vi "Calculate Voltage Array.vi"(1 "I_peak":dbl, 2 "V_min":dbl, 3 "R_ref":dbl, 4 "Scale (True == Linear, False == Log)":bool, 5 "# pts":dbl, 6 "V_max":dbl) -> (0 "Voltage Array":dbl[](array[numeric]))   [LabVIEW 2020]
doc: "Calculate Voltage Array.vi outputs a double numeric array with an inputted number of voltages within an inputted range with an inputted spacing (linear or log). No more voltages are appended to the array when an inputted peak current can theoretically be reached."
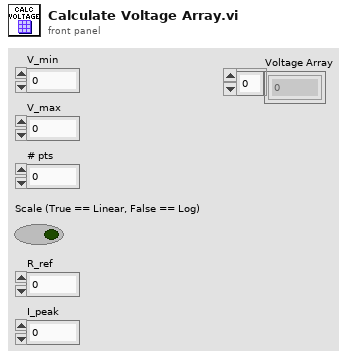
[diagram p1: front panel]
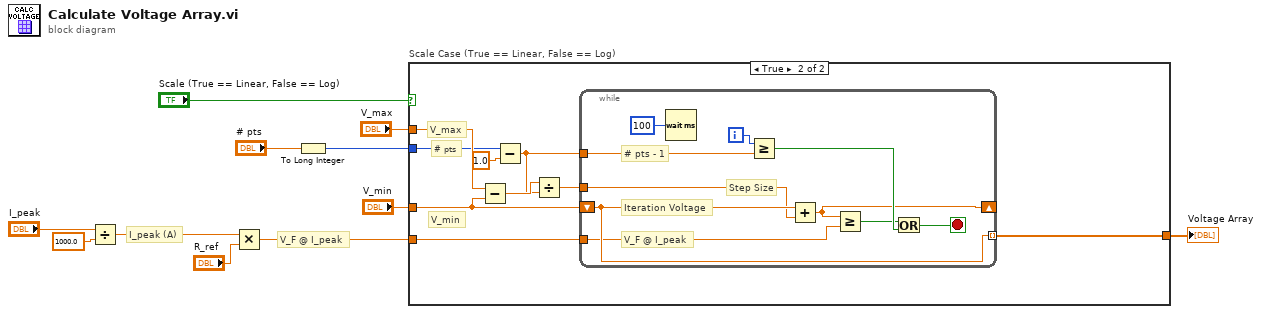
[diagram p0: block diagram]
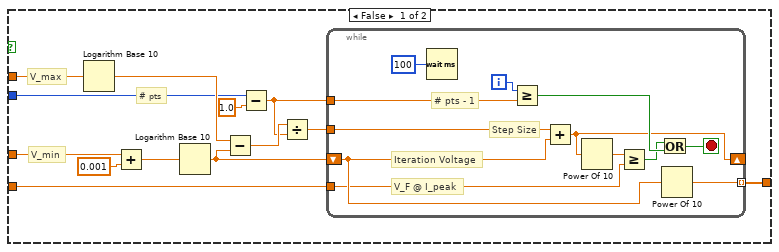
[diagram p2: hidden frame]
diagram:
  # "V_F @ I_peak"
  # "I_peak (A)"
  n1 = Divide(x="I_peak", y=1000.0) -> (x/y=w5:dbl)
  n2 = Multiply(x=w5, y="R_ref") -> (x*y=w2:dbl)
  n3 = To Long Integer(number="# pts") -> (32bit integer=w7:i32)
  n4 = case "Scale Case (True == Linear, False == Log)" shown="True" "Scale (True == Linear, False == Log)" {
    tunnel: [w18 w43] -> w1
    tunnel: "V_min" -> [w16 w39]
    tunnel: "V_max" -> [w15 w41]
    tunnel: w7 -> [w14 w40]
    tunnel: w2 -> [w12 w37]
    frame False {
      # "# pts"
      # "V_min"
      # "V_max"
      n5 = Logarithm Base 10(1:w15) -> (0:w24:dbl)
      n6 = Add(x=w16, y=0.001) -> (x+y=w22:dbl)
      n7 = Logarithm Base 10(1:w22) -> (0:w20:dbl)
      n8 = Subtract(x=w24, y=w20) -> (x-y=w21:dbl)
      n9 = Subtract(x=w14, y=1.0) -> (x-y=w13:dbl)
      n10 = Divide(x=w21, y=w13) -> (x/y=w19:dbl)
      n11 = while {
        shift-right: [w28] -> _
        shift-left: w20 -> [w35]
        tunnel: w19 -> [w36]
        tunnel: [w34] -> w18 mode=indexing
        tunnel: w13 -> [w32]
        tunnel: w12 -> [w25]
        i -> [w33]
        stop <- w29 stop-if-true
        # "V_F @ I_peak"
        # "# pts - 1"
        # "Iteration Voltage"
        # "Step Size"
        n12 = Wait (ms)(milliseconds to wait=u32 100) -> ()  [unwired: 1 out]
        n13 = Greater Or Equal?(x=w33, y=w32) -> (x >= y?=w30:bool)
        n14 = Add(x=w36, y=w35) -> (x+y=w28:dbl)
        n15 = Power Of 10(x=w28) -> (10^x=w27:dbl)
        n16 = Greater Or Equal?(x=w27, y=w25) -> (x >= y?=w26:bool)
        n17 = Or(x=w26, y=w30) -> (x .or. y?=w29:bool)
        n18 = Power Of 10(x=w35) -> (10^x=w34:dbl)
      }
    }
    frame True {
      # "# pts"
      # "V_min"
      # "V_max"
      n19 = Subtract(x=w41, y=w39) -> (x-y=w45:dbl)
      n20 = Subtract(x=w40, y=1.0) -> (x-y=w38:dbl)
      n21 = Divide(x=w45, y=w38) -> (x/y=w44:dbl)
      n22 = while {
        tunnel: w44 -> [w51]
        shift-right: [w47] -> _
        shift-left: w39 -> [w55]
        tunnel: [w55] -> w43 mode=indexing
        tunnel: w38 -> [w53]
        tunnel: w37 -> [w46]
        i -> [w54]
        stop <- w48 stop-if-true
        # "# pts - 1"
        # "V_F @ I_peak"
        # "Step Size"
        # "Iteration Voltage"
        n23 = Wait (ms)(milliseconds to wait=u32 100) -> ()  [unwired: 1 out]
        n24 = Greater Or Equal?(x=w54, y=w53) -> (x >= y?=w50:bool)
        n25 = Add(x=w55, y=w51) -> (x+y=w47:dbl)
        n26 = Greater Or Equal?(x=w47, y=w46) -> (x >= y?=w49:bool)
        n27 = Or(x=w49, y=w50) -> (x .or. y?=w48:bool)
      }
    }
  }
  "Voltage Array" <- w1
